vi "SetPulWidth.vi"(8 "错误输入（无错误）":errorcluster, 10 "采样脉冲宽度":u32) -> (0 "错误输出":errorcluster)   [LabVIEW 2018]
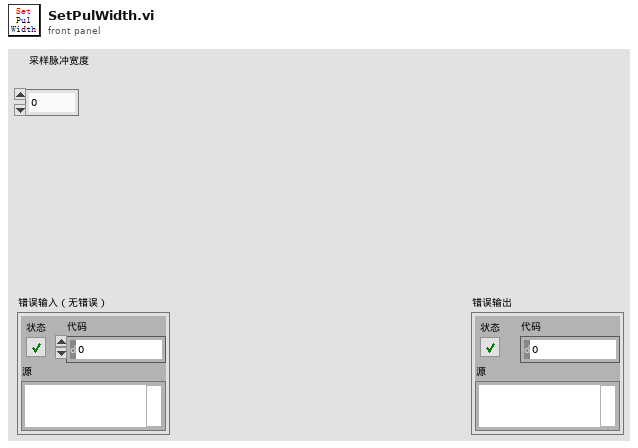
[diagram p1: front panel]
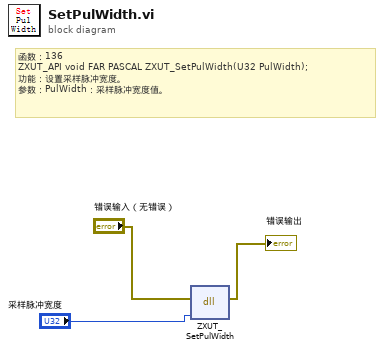
[diagram p0: block diagram]
diagram:
  # "函数：136\nZXUT_API void\tFAR PASCAL ZXUT_SetPulWidth(U32 PulWidth);\n功能：设置采样脉冲宽度。\n参数：PulWidth：采样脉冲宽度值。"
  n1 = dll-call lib="PTH2Rabs E软件项目超声超声子VI函数VI\tTCG处理ZXUTConfigMgr.dll" fn="ZXUT_SetPulWidth"(error in="错误输入（无错误）", "PulWidth"="采样脉冲宽度") -> (error out=→"错误输出":errorcluster)  [unwired: 4 in, 1 out]
